vi "6_1.vi"() -> ()   [LabVIEW 2021, in "2023.lvlib"]
uses:
  2023.lvlib
panel:
  out "Result":i32
  in  "Demo / Real Input":bool
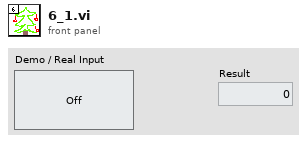
[diagram p1: front panel]
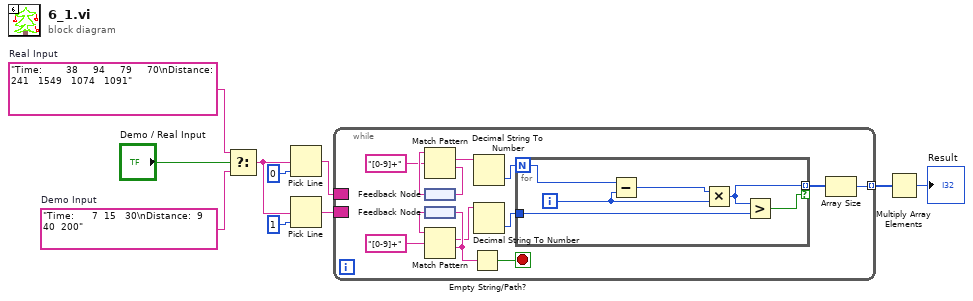
[diagram p0: block diagram]
diagram:
  w10 = "Time:        38     94     79     70\nDistance:   241   1549   1074   1091"  # Real Input
  w9 = "Time:      7  15   30\nDistance:  9  40  200"  # Demo Input
  n1 = Select(t=w10, s="Demo / Real Input", f=w9) -> (s? t:f=w7:string)
  n2 = Pick Line(multi-line string=w7, line index=0) -> (output string=w4:string)  [unwired: 1 in]
  n3 = Pick Line(multi-line string=w7, line index=1) -> (output string=w3:string)  [unwired: 1 in]
  n4 = while {
    border: w4 -> [_]
    border: w3 -> [_]
    tunnel: [w11] -> w2 mode=indexing
    stop <- w23 stop-if-true
    n5 = feedback #1() -> (w22:string)
    n6 = Match Pattern(string=w22, regular expression="[0-9]+" ("format string")) -> (match substring=w17:string, after substring=w16:string)  [unwired: 1 in, 2 out]
    n7 = feedback-in #1(w16) -> ()
    n8 = feedback #2() -> (w20:string)
    n9 = Match Pattern(string=w20, regular expression="[0-9]+" ("format string")) -> (match substring=w15:string, after substring=w18:string)  [unwired: 1 in, 2 out]
    n10 = feedback-in #2(w18) -> ()
    n11 = Empty String/Path?(string/path=w18) -> (empty?=w23:bool)
    n12 = Decimal String To Number(string=w17) -> (number=w14:i32)  [unwired: 2 in, 1 out]
    n13 = Decimal String To Number(string=w15) -> (number=w13:i32)  [unwired: 2 in, 1 out]
    n14 = for {
      N: w14 -> [w29]
      tunnel: [w26] -> w12 mode=indexing if=w24
      tunnel: w13 -> [w25]
      i -> [w27]
      n15 = Subtract(x=w29, y=w27) -> (x-y=w28:i32)
      n16 = Multiply(x=w28, y=w27) -> (x*y=w26:i32)
      n17 = Greater?(x=w26, y=w25) -> (0:w24:bool)
    }
    n18 = Array Size(array=w12) -> (size(s)=w11:i32)
  }
  n19 = Multiply Array Elements(1:w2) -> (0:→"Result":i32)
